vi "test Loopback RT to BC.vi"(8 "error in":errorcluster, 11 "TestCase in":refnum<class "Loopback.lvclass">) -> (0 "error out":errorcluster, 3 "TestCase out":refnum<class "Loopback.lvclass">)   [LabVIEW 2020, in "Loopback.lvclass"]
uses:
  Loopback.lvclass
  C:/dev/niveristand-custom-device-testing-tools/VeriStandTestCase/VeriStandTestCase.lvclass
  <vilib>/numeric/Random Number (Range) U64.vi
  485b7c2b-8320-4722-9ec7-d01f27c65546.vi
  <vilib>/numeric/sub_Random U32.vi
  <vilib>/NI VeriStand/Execution/Workspace/NI VeriStand - Set Multiple Channel Values.vi
  <vilib>/NI VeriStand/Execution/Workspace/NI VeriStand - Get Multiple Channel Values.vi
  <vilib>/addons/_JKI Toolkits/VI Tester/TestCase.llb/TestCase.lvclass
  <vilib>/NI VeriStand/Execution/Workspace/NI_VS Workspace ExecutionAPI.lvlib
  C:/Program Files (x86)/National Instruments/LabVIEW 2020/vi.lib/addons/_JKI Toolkits/VI Tester/TestCase.llb/TestCase.lvclass
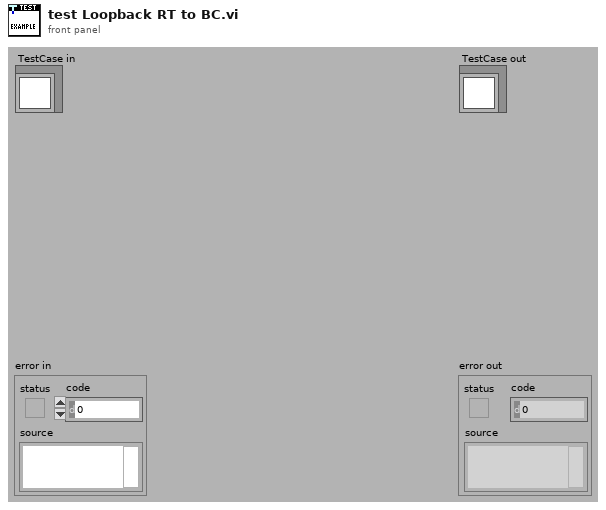
[diagram p1: front panel]
types:
  T1 = typedef "NI_VS Workspace ExecutionAPI.lvlib/WorkspaceAPI.ctl" = refnum<k24>
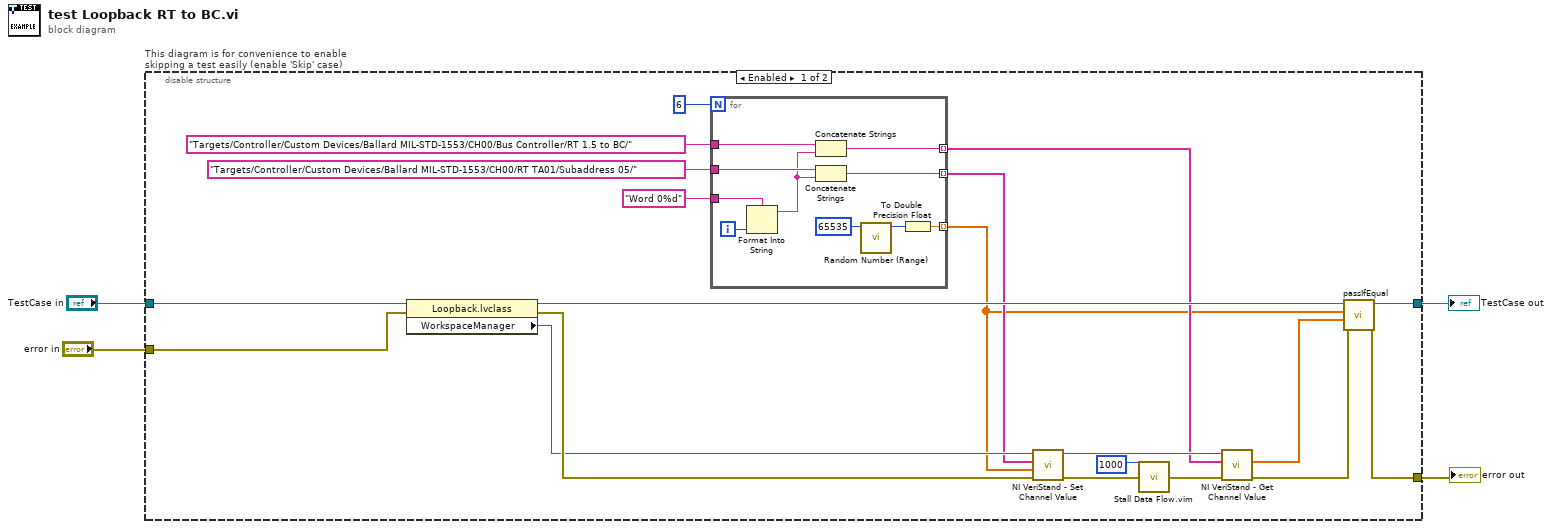
[diagram p0: block diagram]
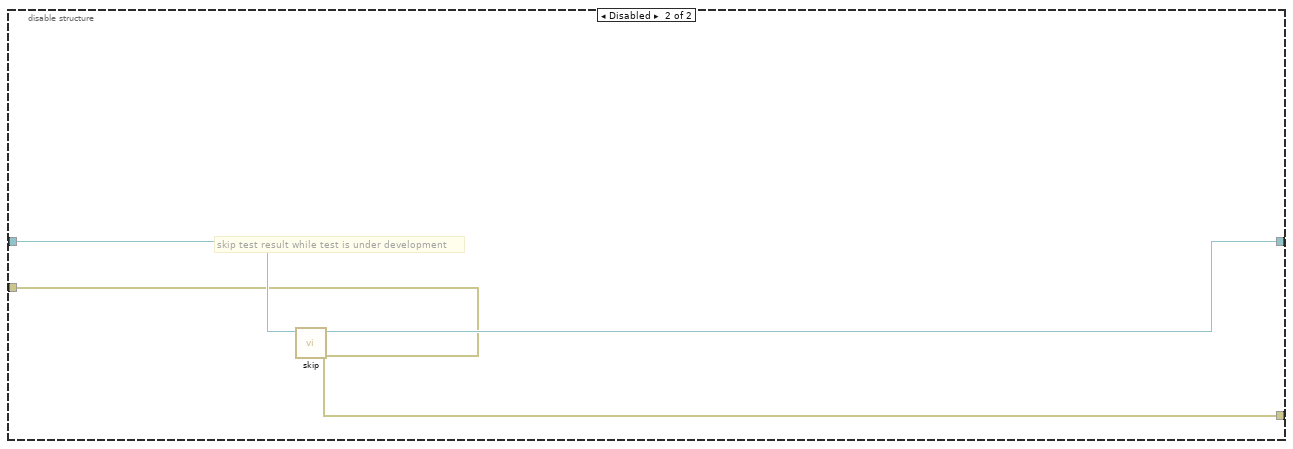
[diagram p2: hidden frame]
diagram:
  n1 = disable-structure "This diagram is for convenience to enable skipping a test easily (enable 'Skip' case)" shown="Enabled" {
    disable-tunnel: "TestCase in" -> [w14 w38]
    disable-tunnel: [w16 w36] -> w1
    disable-tunnel: [w8 w37] -> w3
    disable-tunnel: "error in" -> [w9 w35]
    frame Enabled {
      n2 = property class="Loopback.lvclass"(reference=w14, error in=w9) -> (reference out=w24:refnum<class "Loopback.lvclass">, error out=w19:errorcluster, "WorkspaceManager"=w17:T1)
      n3 = for {
        N: 6 -> [_]
        tunnel: "Targets/Controller/Custom Devices/Ballard MIL-STD-1553/CH00/RT TA01/Subaddress 05/" ("Channel") -> [w33]
        tunnel: [w34] -> w12 mode=indexing
        tunnel: "Targets/Controller/Custom Devices/Ballard MIL-STD-1553/CH00/Bus Controller/RT 1.5 to BC/" ("Channel") -> [w32]
        tunnel: [w31] -> w10 mode=indexing
        tunnel: "Word 0%d" -> [w29]
        tunnel: [w25] -> w5 mode=indexing
        i -> [w30]
        n4 = Format Into String(format string=w29, w30) -> (resulting string=w28:string)  [unwired: 2 in, 1 out]
        n5 = Concatenate Strings(w32, w28) -> (w31:string)
        n6 = Concatenate Strings(w33, w28) -> (w34:string)
        n7 = call-poly <vilib>:"Random Number (Range).vi"("upper bound (100)"=u64 65535) -> ("number"=w27:u64)  [unwired: 10 in]
        n8 = To Double Precision Float(number=w27) -> (double precision float=w25:dbl)
      }
      n9 = call-poly <vilib>:"NI VeriStand - Set Channel Value.vi"("error in (no error)"=w19, "Values"=w5, "Channels"=w12, "WorkspaceManager in"=w17) -> ("error out"=w21:errorcluster, "WorkspaceManager out"=w23:T1)  [unwired: 6 in]
      n10 = call "Stall Data Flow.vim"("value in"=w21, "milliseconds to wait"=u32 1000) -> ("value out"=w22:errorcluster)  [unwired: 1 out]
      n11 = call-poly <vilib>:"NI VeriStand - Get Channel Value.vi"("error in (no error)"=w22, "Channels"=w10, "WorkspaceManager in"=w23) -> ("error out"=w18:errorcluster, "Values"=w15:dbl[])  [unwired: 6 in, 1 out]
      n12 = call-dynamic "passIfEqual.vi"("error in (no error)"=w18, "y"=w15, "x"=w5, "TestCase in"=w24) -> ("error out"=w8:errorcluster, "TestCase out"=w16:refnum<class "Loopback.lvclass">)  [unwired: 6 in]
    }
    frame Disabled {
      # "skip test result while test is under development"
      n13 = call <vilib>:"skip.vi"("error in (no error)"=w35, "TestCase in"=w38) -> ("error out"=w37:errorcluster, "TestCase out"=w36:refnum<class "Loopback.lvclass">)  [unwired: 8 in]
    }
  }
  "error out" <- w3
  "TestCase out" <- w1
